vi "Initialize Attributes.vi"(8 "error in (no error)":errorcluster, 10 "Attribute Data":variant, 11 "CS++DeviceActor in":refnum<class "CS++DeviceActor.lvclass">) -> (0 "error out":errorcluster, 2 "Found?":bool, 3 "CS++DeviceActor out":refnum<class "CS++DeviceActor.lvclass">)   [LabVIEW 2014, in "CS++DeviceActor.lvlib" / "CS++DeviceActor.lvclass"]
doc: "Initialize object attribute.\n\nUnique resources should be allocated elsewhere!"
uses:
  CS++DeviceActor.lvclass
  Classes/CS++ProcessVariables/ProcessVariable/PV.lvclass
  CS++BaseActor/CS++BaseActor.lvclass/CS++BaseActor.ctl
  Classes/CS++ProcessVariables/ProcessVariable/PV.lvclass/PV.ctl
  CS++DeviceActor.lvclass/CS++DeviceActor.ctl
  Classes/CS++ProcessVariables/ProcessVariable/Write Name.vi
  Classes/CS++ProcessVariables/ProcessVariable/Write PV URL.vi
  Classes/CS++ProcessVariables/ProcessVariable/Write Type Descriptor.vi
  CS++BaseActor/CS++BaseActor.lvclass
  Classes/CS++BaseClasses/Factory/CS++Factory.lvclass
  Classes/CS++ProcessVariables/CS++ProcessVariables.lvlib
  Libraries/Utilities/CS++Utilities.lvlib
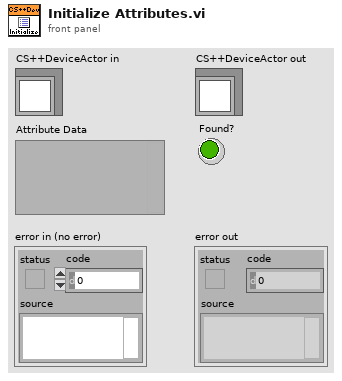
[diagram p1: front panel]
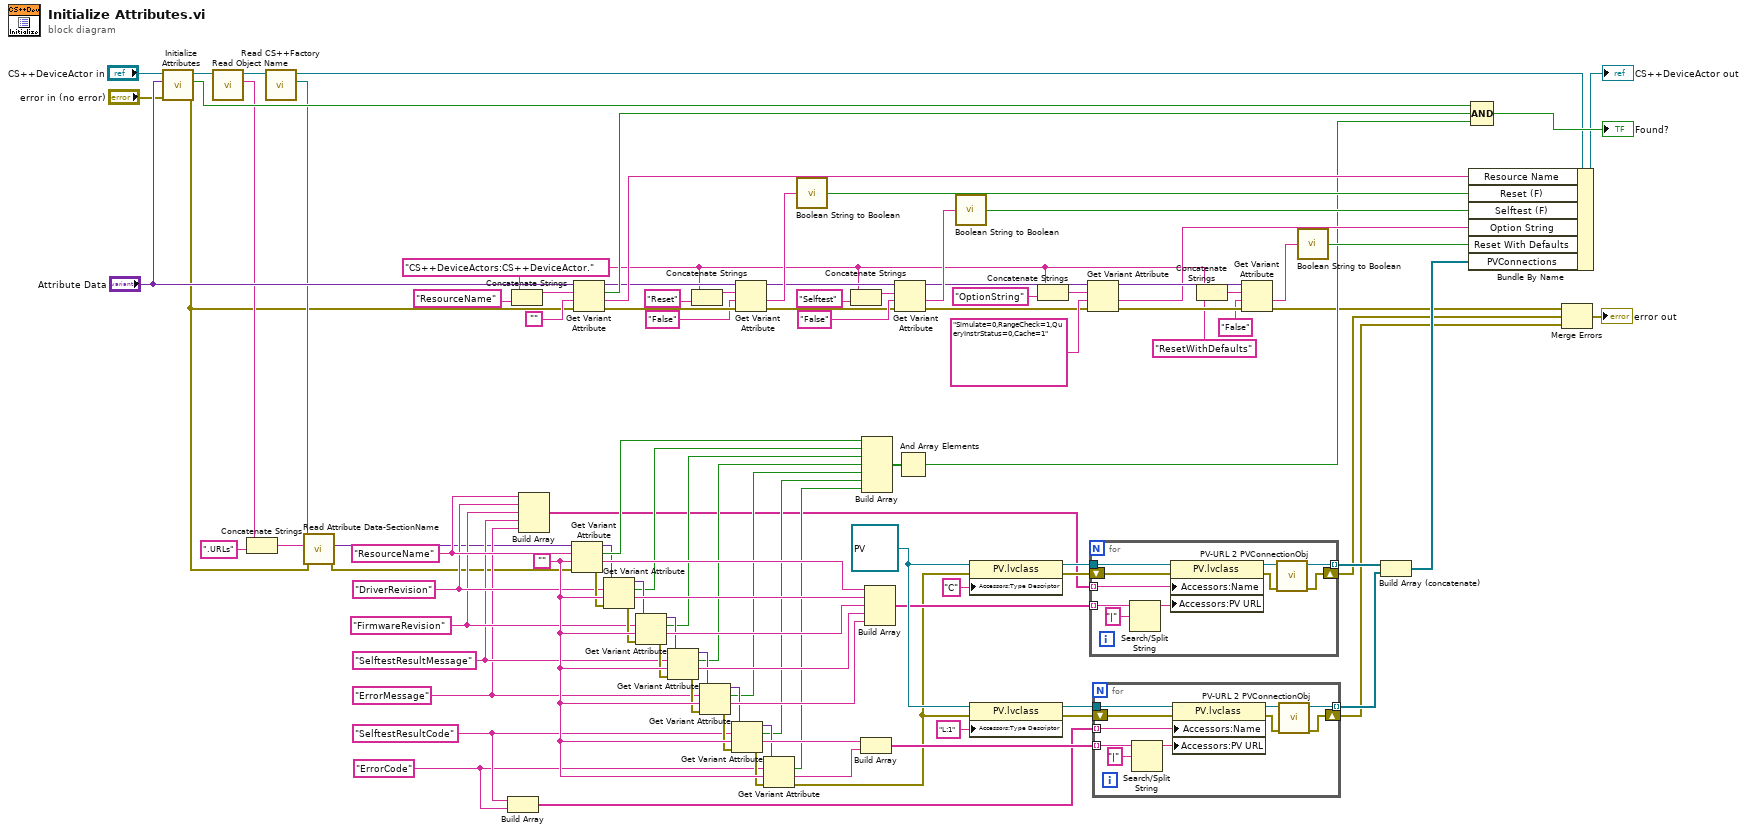
[diagram p0: block diagram]
diagram:
  w59 = refnum<class "PV.lvclass"> refnum ("CS++ProcessVariables.lvlib:PV.lvclass")
  w11 = "ErrorMessage"
  w8 = "ErrorCode"
  w12 = "SelftestResultMessage"
  w9 = "SelftestResultCode"
  w13 = "FirmwareRevision"
  w14 = "DriverRevision"
  w39 = ""
  w15 = "ResourceName"
  w62 = "CS++DeviceActors:CS++DeviceActor."
  n1 = call-parent "Initialize Attributes.vi"("error in (no error)"="error in (no error)", "Attribute Data"="Attribute Data", "CS++BaseActor in"="CS++DeviceActor in") -> ("error out"=w3:errorcluster, "Found?"=w104:bool, "CS++BaseActor out"=w77:refnum<class "CS++DeviceActor.lvclass">)  [unwired: 6 in]
  n2 = call "Read Object Name.vi"("CS++BaseActor in"=w77) -> ("Object Name"=w80:string, "CS++BaseActor out"=w81:refnum<class "CS++DeviceActor.lvclass">)  [unwired: 8 in, 1 out]
  n3 = Concatenate Strings(w80, ".URLs" ("string")) -> (w4:string)
  n4 = call "Read CS++Factory.vi"("CS++BaseActor in"=w81) -> ("CS++Factory"=w5:refnum<class "CS++Factory.lvclass">, "CS++BaseActor out"=w57:refnum<class "CS++DeviceActor.lvclass">)  [unwired: 8 in, 1 out]
  n5 = call-dynamic "Read Attribute Data-SectionName.vi"("error in (no error)"=w3, "Object Name"=w4, "CS++Factory in"=w5) -> ("error out"=w2:errorcluster, "Attribute Data"=w1:variant)  [unwired: 6 in, 1 out]
  n6 = Build Array(w9, w8) -> (w7:string[])
  n7 = Concatenate Strings(w62, "ResourceName") -> (w103:string)
  n8 = Build Array(w15, w14, w13, w12, w11) -> (w10:string[])
  n9 = Get Variant Attribute(Variant=w1, name=w15, default value (empty Variant)=w39, error in=w2) -> (duplicate Variant=w30:variant, found=w31:bool, value=w56:string, error out=w38:errorcluster)
  n10 = Get Variant Attribute(Variant="Attribute Data", name=w103, default value (empty Variant)="", error in=w3) -> (duplicate Variant=w95:variant, found=w98:bool, value=w100:string, error out=w94:errorcluster)
  n11 = Get Variant Attribute(Variant=w30, name=w14, default value (empty Variant)=w39, error in=w38) -> (duplicate Variant=w29:variant, found=w24:bool, value=w55:string, error out=w37:errorcluster)
  n12 = Get Variant Attribute(Variant=w29, name=w13, default value (empty Variant)=w39, error in=w37) -> (duplicate Variant=w28:variant, found=w23:bool, value=w54:string, error out=w36:errorcluster)
  n13 = Get Variant Attribute(Variant=w28, name=w12, default value (empty Variant)=w39, error in=w36) -> (duplicate Variant=w27:variant, found=w22:bool, value=w53:string, error out=w35:errorcluster)
  n14 = Concatenate Strings(w62, "Reset") -> (w96:string)
  n15 = Get Variant Attribute(Variant=w27, name=w11, default value (empty Variant)=w39, error in=w35) -> (duplicate Variant=w26:variant, found=w21:bool, value=w52:string, error out=w34:errorcluster)
  n16 = Get Variant Attribute(Variant=w26, name=w9, default value (empty Variant)=w39, error in=w34) -> (duplicate Variant=w25:variant, found=w20:bool, value=w48:string, error out=w33:errorcluster)
  n17 = Get Variant Attribute(Variant=w95, name=w96, default value (empty Variant)="False", error in=w94) -> (duplicate Variant=w87:variant, value=w92:string, error out=w82:errorcluster)  [unwired: 1 out]
  n18 = Get Variant Attribute(Variant=w25, name=w8, default value (empty Variant)=w39, error in=w33) -> (found=w19:bool, value=w47:string, error out=w32:errorcluster)  [unwired: 1 out]
  n19 = call "Boolean String to Boolean.vi"("T/F String"=w92) -> ("Value"=w91:bool)
  n20 = Concatenate Strings(w62, "Selftest") -> (w89:string)
  n21 = Build Array(w48, w47) -> (w46:string[])
  n22 = Build Array(w31, w24, w23, w22, w21, w20, w19) -> (w18:bool[])
  n23 = Build Array(w56, w55, w54, w53, w52) -> (w51:string[])
  n24 = Get Variant Attribute(Variant=w87, name=w89, default value (empty Variant)="False", error in=w82) -> (duplicate Variant=w66:variant, value=w86:string, error out=w63:errorcluster)  [unwired: 1 out]
  n25 = And Array Elements(Boolean array=w18) -> (logical AND=w17:bool)
  n26 = call "Boolean String to Boolean.vi"("T/F String"=w86) -> ("Value"=w85:bool)
  n27 = property class="PV.lvclass"(reference=w59, error in=w32, "Accessors:Type Descriptor"="C" ("Type Descriptor")) -> (reference out=w58:refnum<class "PV.lvclass">, error out=w50:errorcluster)
  n28 = property class="PV.lvclass"(reference=w59, error in=w32, "Accessors:Type Descriptor"="L:1" ("Type Descriptor")) -> (reference out=w49:refnum<class "PV.lvclass">, error out=w6:errorcluster)
  n29 = Concatenate Strings(w62, "OptionString" ("string")) -> (w75:string)
  n30 = Get Variant Attribute(Variant=w66, name=w75, default value (empty Variant)="Simulate=0,RangeCheck=1,QueryInstrStatus=0,Cache=1" ("string"), error in=w63) -> (duplicate Variant=w71:variant, value=w64:string, error out=w72:errorcluster)  [unwired: 1 out]
  n31 = for {
    tunnel: w58 -> [w113]
    tunnel: w51 -> [w107] mode=indexing
    tunnel: [w112] -> w45 mode=indexing
    shift-right: [w111] -> w42
    shift-left: w50 -> [w109]
    tunnel: w10 -> [w108] mode=indexing
    n32 = Search/Split String(string=w107, search string/char (-)="|") -> (substring before match=w106:string)  [unwired: 1 in, 2 out]
    n33 = property class="PV.lvclass"(reference=w113, error in=w109, "Accessors:Name"=w108, "Accessors:PV URL"=w106) -> (reference out=w114:refnum<class "PV.lvclass">, error out=w110:errorcluster)
    n34 = call "PV-URL 2 PVConnectionObj.vi"("Error In"=w110, "PV"=w114) -> ("Error Out"=w111:errorcluster, "PVConnection"=w112:refnum<class "PVConnection.lvclass">)  [unwired: 7 in, 1 out]
  }
  n35 = for {
    tunnel: w49 -> [w123]
    tunnel: w46 -> [w116] mode=indexing
    tunnel: [w122] -> w44 mode=indexing
    shift-right: [w121] -> w41
    shift-left: w6 -> [w119]
    tunnel: w7 -> [w118] mode=indexing
    n36 = Search/Split String(string=w116, search string/char (-)="|") -> (substring before match=w115:string)  [unwired: 1 in, 2 out]
    n37 = property class="PV.lvclass"(reference=w123, error in=w119, "Accessors:Name"=w118, "Accessors:PV URL"=w115) -> (reference out=w124:refnum<class "PV.lvclass">, error out=w120:errorcluster)
    n38 = call "PV-URL 2 PVConnectionObj.vi"("Error In"=w120, "PV"=w124) -> ("Error Out"=w121:errorcluster, "PVConnection"=w122:refnum<class "PVConnection.lvclass">)  [unwired: 7 in, 1 out]
  }
  n39 = Concatenate Strings(w62, "ResetWithDefaults" ("string")) -> (w70:string)
  n40 = Get Variant Attribute(Variant=w71, name=w70, default value (empty Variant)="False" ("string"), error in=w72) -> (value=w68:string, error out=w16:errorcluster)  [unwired: 2 out]
  n41 = call "Boolean String to Boolean.vi"("T/F String"=w68) -> ("Value"=w65:bool)
  n42 = Build Array (concatenate)(w45, w44) -> (w43:refnum<class "PVConnection.lvclass">[])
  n43 = Bundle By Name(cluster=w57, "Resource Name"=w100, "Reset (F)"=w91, "Selftest (F)"=w85, "Option String"=w64, "Reset With Defaults"=w65, "PVConnections"=w43) -> (→"CS++DeviceActor out":refnum<class "CS++DeviceActor.lvclass">)
  n44 = Compound Arithmetic op=AND(w104, w98, w17) -> (→"Found?":bool)
  n45 = Merge Errors(w16, w42, w41) -> (→"error out":errorcluster)
